vi "rpm_2_torquesetpoints.vi"(0 "C_d":dbl=0.35, 1 "Density_Air(kg/m^3)":dbl=1.225, 2 "Frontal Area(m^2)":dbl=3.5, 3 "Slope(degrees)":dbl, 4 "Mass(kg)":dbl=1800.0, 5 "derivative":dbl, 7 "Gravitational accelaration(m/s^2)":dbl=9.81, 9 "Rolling Resistance Coefficient C_rf":dbl=0.008, 10 "RPM":dbl=542.1878074407578, 11 "Tyre Diameter(m)":dbl=0.5) -> (12 "C1":dbl=0.7503125, 13 "C2":dbl=141.264, 14 "D1":dbl=0.00012856402000333957, 15 "Torque Setpoints_graph":dbl=79.4971584126854, 16 "D2":dbl=35.316, 17 "D3":dbl=11.780972450961723, 18 "dx/dt":dbl format="%0.2f", 19 "C3":dbl=1800.0)   [LabVIEW 2019]
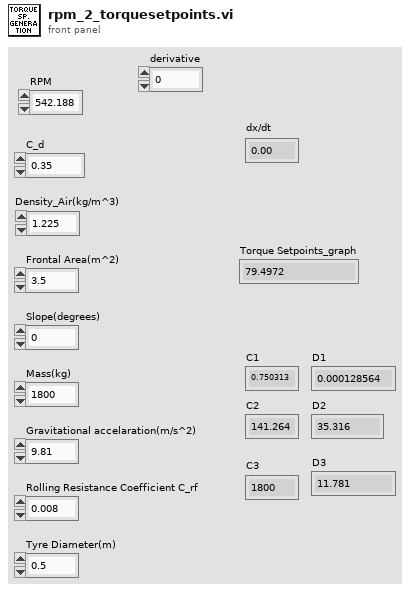
[diagram p1: front panel]
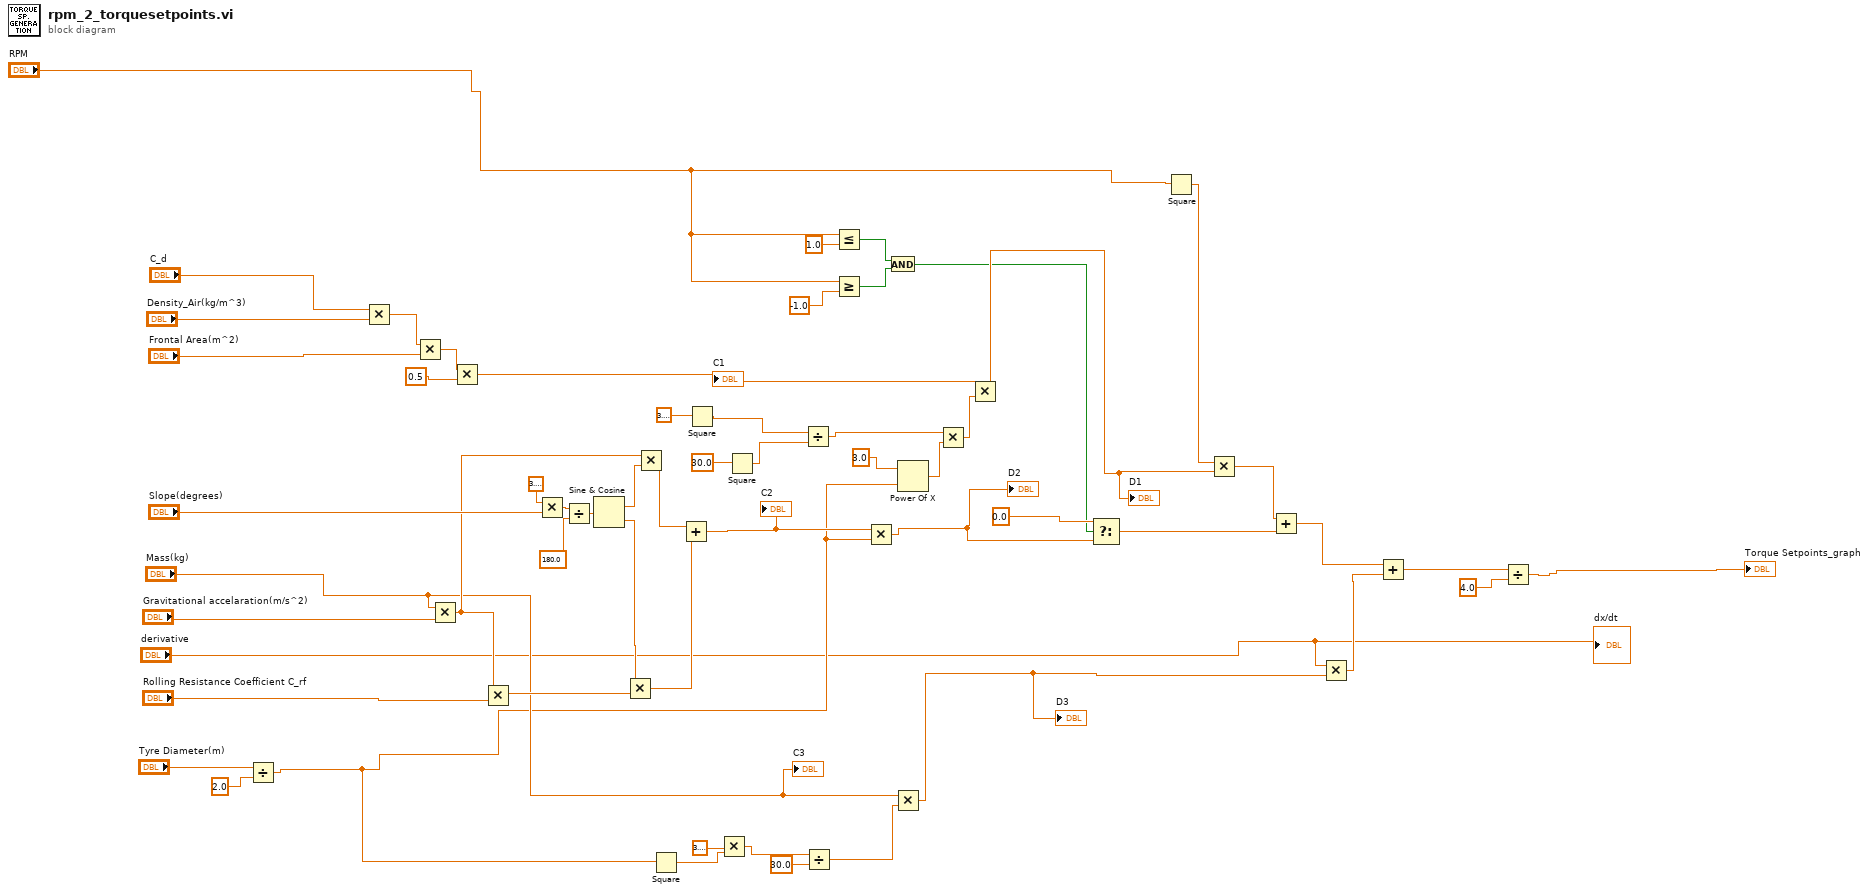
[diagram p0: block diagram]
diagram:
  n1 = Divide(x="Tyre Diameter(m)", y=2.0) -> (x/y=w6:dbl)
  n2 = Multiply(x="C_d", y="Density_Air(kg/m^3)") -> (x*y=w37:dbl)
  n3 = Multiply(x=w37, y="Frontal Area(m^2)") -> (x*y=w39:dbl)
  n4 = Multiply(x="Mass(kg)", y="Gravitational accelaration(m/s^2)") -> (x*y=w45:dbl)
  n5 = Multiply(x=w39, y=0.5 ("x*y")) -> (x*y=w54:dbl)
  "C1" <- w54
  n6 = Multiply(x=w45, y="Rolling Resistance Coefficient C_rf") -> (x*y=w43:dbl)
  n7 = Multiply(x=3.141592653589793, y="Slope(degrees)") -> (x*y=w51:dbl)
  n8 = Divide(x=w51, y=180.0 ("x/y")) -> (x/y=w53:dbl)
  n9 = Sine & Cosine(0:w53) -> (1:w46:dbl, 2:w44:dbl)
  n10 = Multiply(x=w44, y=w43) -> (x*y=w48:dbl)
  n11 = Multiply(x=w45, y=w46) -> (x*y=w47:dbl)
  n12 = Square(x=w6) -> (x^2=w22:dbl)
  n13 = Add(x=w47, y=w48) -> (x+y=w24:dbl)
  "C2" <- w24
  n14 = Square(x=3.141592653589793) -> (x^2=w33:dbl)
  n15 = Multiply(x=3.141592653589793, y=w22) -> (x*y=w21:dbl)
  n16 = Square(x=30.0 ("y")) -> (x^2=w30:dbl)
  n17 = Divide(x=w33, y=w30) -> (x/y=w29:dbl)
  n18 = Divide(x=w21, y=30.0) -> (x/y=w18:dbl)
  n19 = Less Or Equal?(x="RPM", y=1.0) -> (x <= y?=w11:bool)
  n20 = Greater Or Equal?(x="RPM", y=-1.0) -> (x >= y?=w10:bool)
  n21 = Multiply(x=w24, y=w6) -> (x*y=w16:dbl)
  "D2" <- w16
  n22 = And(x=w11, y=w10) -> (x .and. y?=w9:bool)
  n23 = Multiply(x="Mass(kg)", y=w18) -> (x*y=w17:dbl)
  "D3" <- w17
  n24 = Power Of X(1:w6, 2:3.0 ("x^y")) -> (0:w27:dbl)
  n25 = Multiply(x=w29, y=w27) -> (x*y=w28:dbl)
  n26 = Multiply(x=w54, y=w28) -> (x*y=w34:dbl)
  "D1" <- w34
  n27 = Select(t=0.0, s=w9, f=w16) -> (s? t:f=w15:dbl)
  n28 = Square(x="RPM") -> (x^2=w8:dbl)
  n29 = Multiply(x=w8, y=w34) -> (x*y=w55:dbl)
  n30 = Add(x=w55, y=w15) -> (x+y=w56:dbl)
  n31 = Multiply(x="derivative", y=w17) -> (x*y=w57:dbl)
  n32 = Add(x=w56, y=w57) -> (x+y=w3:dbl)
  n33 = Divide(x=w3, y=4.0) -> (x/y=→"Torque Setpoints_graph":dbl)
  "C3" <- "Mass(kg)"
  "dx/dt" <- "derivative"
